vi "Compostite Employee.vi"(0 "Composite Employee in":refnum<class "Composite Employee.lvclass">, 5 "name":string, 7 "dept":string, 9 "sal":string, 11 "error in (no error)":errorcluster) -> (4 "Composite Employee out":refnum<class "Composite Employee.lvclass">, 15 "error out":errorcluster)   [LabVIEW 2017, in "Composite Employee.lvclass"]
uses:
  Composite Employee.lvclass
  Composite Employee.lvclass/Composite Employee.ctl
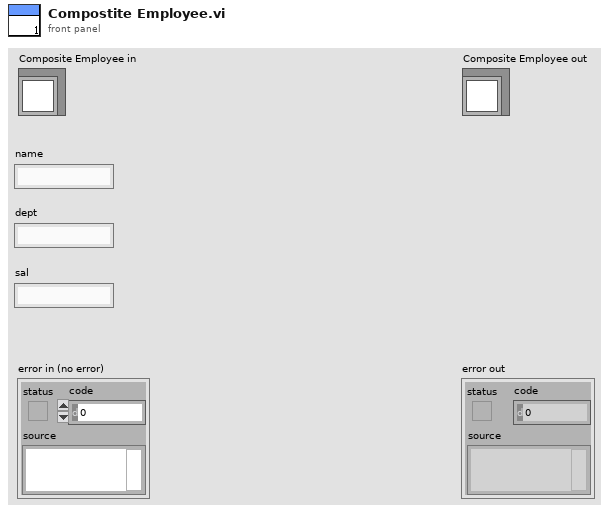
[diagram p1: front panel]
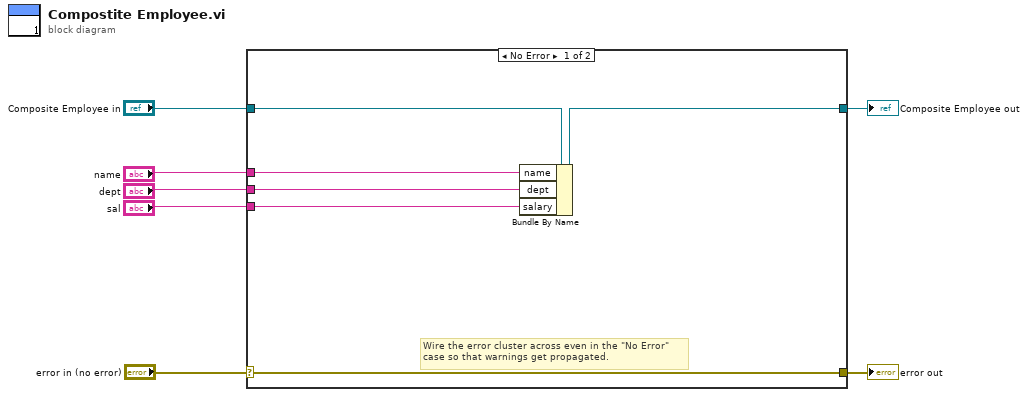
[diagram p0: block diagram]
diagram:
  n1 = case shown="No Error" "error in (no error)" {
    selector: "error in (no error)" -> [w12 w15]
    tunnel: [w12 w15] -> w6
    tunnel: [w11 w14] -> w4
    tunnel: "Composite Employee in" -> [w13 w14]
    tunnel: "name" -> [w10 _]
    tunnel: "dept" -> [w9 _]
    tunnel: "sal" -> [w8 _]
    frame No Error {
      # "Wire the error cluster across even in the \"No Error\"\ncase so that warnings get propagated."
      n2 = Bundle By Name(cluster=w13, "name"=w10, "dept"=w9, "salary"=w8) -> (w11:refnum<class "Composite Employee.lvclass">)
    }
    frame Error {
    }
  }
  "error out" <- w6
  "Composite Employee out" <- w4
